vi "FTW-Logger-WriteFile.vi"(0 "FTW Logger":refnum<class "FTW-Logger-Instance.lvclass">, 5 "Entries to Log":string[](array[string]), 11 "error in":errorcluster) -> (4 "FTW Logger out":refnum<class "FTW-Logger-Instance.lvclass">, 15 "error out":errorcluster)   [LabVIEW 2013, in "FTW-Logger-Instance.lvclass"]
uses:
  FTW-Logger-Instance.lvclass
  FTW-Logger-Instance.lvclass/FTW-Logger-Instance.ctl
panel:
  # "Inputs"
  # "Outputs"
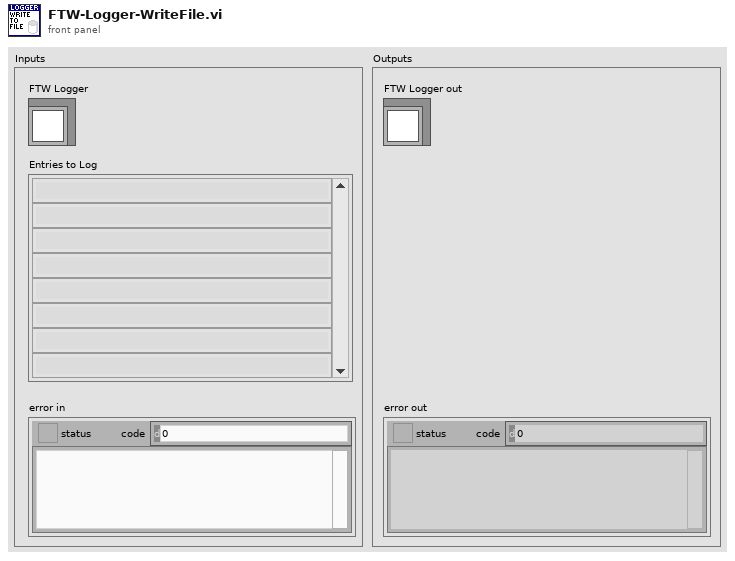
[diagram p1: front panel]
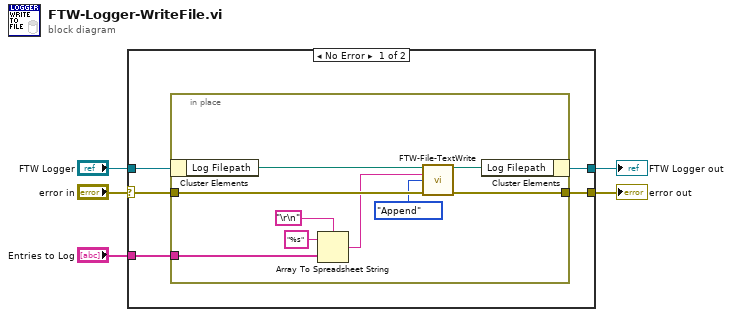
[diagram p0: block diagram]
diagram:
  n1 = case shown="No Error" "error in" {
    selector: "error in" -> [w8 w21]
    tunnel: [w7 w21] -> w2
    tunnel: [w9 w20] -> w4
    tunnel: "FTW Logger" -> [w10 w20]
    tunnel: "Entries to Log" -> [w6 _]
    frame No Error {
      n2 = in-place {
        in-place-border: w6 -> [w15]
        in-place-border: w8 -> [w17]
        in-place-border: [w16] -> w7
        n3 = in-place-cluster #1(w10) -> ("Log Filepath"=w19:path)
        n4 = Array To Spreadsheet String(delimiter (Tab)="\r\n", array=w15, 3:"%s" ("format string")) -> (spreadsheet string=w14:string)
        n5 = call "FTW-File-TextWrite.vi"("Filepath"=w19, "Text to Write"=w14, "Mode"=enum16{"Overwrite", "Append"}."Append", "error in"=w17) -> ("Filepath out"=w18:path, "error out"=w16:errorcluster)  [unwired: 10 in]
        n6 = in-place-cluster #1("Log Filepath"=w18) -> (w9:refnum<class "FTW-Logger-Instance.lvclass">)
      }
    }
    frame Error {
    }
  }
  "error out" <- w2
  "FTW Logger out" <- w4
